vi "Periodic Tasks.vi"   [LabVIEW 2015]
doc: "This VI runs in parallel to other robot code. It can contain as many user-defined periodic loops as you need. These can carry out PID or other sorts of timed response."
uses:
  <vilib>/Rock Robotics/Network Tables/NT Read Boolean.vi
  Robot Global Data.vi
  <vilib>/Rock Robotics/Network Tables/NT Write Boolean.vi
  <vilib>/Rock Robotics/Network Tables/NT Write Number.vi
  Support Code/Team900-VIs/navX Library v2/navX Library v2.lvlib
types:
  T1 = typedef "navX Library v2.lvlib/Z900_navX_DeviceTypeDef.ctl" = cluster{"Interface":cluster{"Protocol":T2, "Update Rate (4Hz-60Hz)":u8, "navX Open TypeDef":variant}, "Notify Packet":refnum<notifier>, "Loop VI Refnum":refnum<vi>, "Ready to Close Occurrence Refnum":refnum<k4>}
  T2 = typedef "navX Library v2.lvlib/Z900_navX_ProtocolTypeDef.ctl" = enum16{"SERIAL", "I2C", "SPI"}
  T3 = cluster{"Yaw":dbl, "Roll":dbl, "Pitch":dbl, "Heading":dbl, "Fused Heading":dbl}
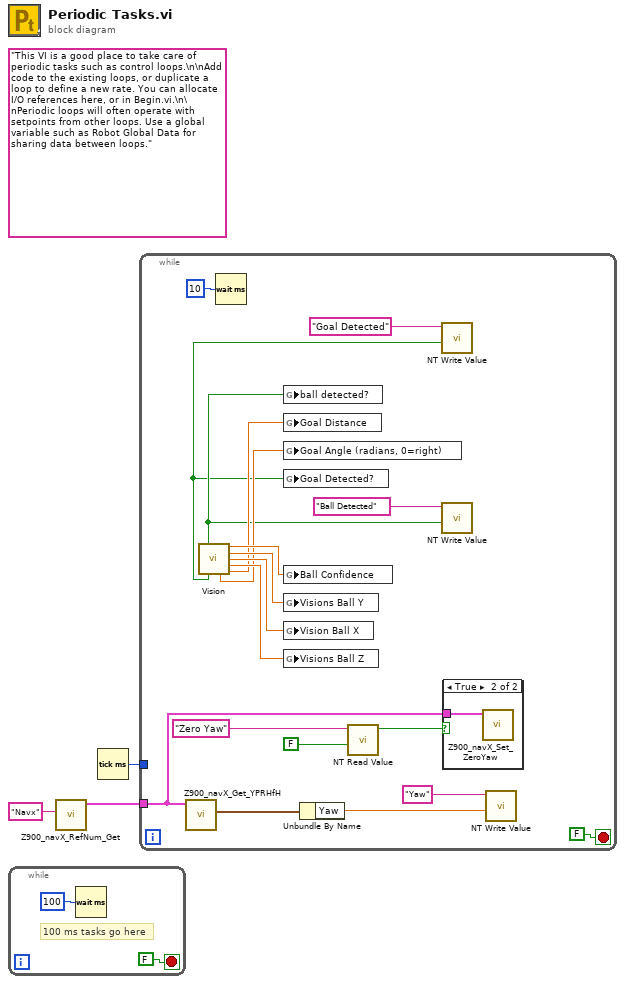
[diagram p0: block diagram]
diagram:
  (unwired) "This VI is a good place to take care of periodic tasks such as control loops.\n\nAdd code to the existing loops, or duplicate a loop to define a new rate. You can allocate I/O references here, or in Begin.vi.\n\nPeriodic loops will often operate with setpoints from other loops. Use a global variable such as Robot Global Data for sharing data between loops."
  n1 = while {
    stop <- FALSE stop-if-true
    # "100 ms tasks go here"
    n2 = Wait (ms)(milliseconds to wait=u32 100) -> ()  [unwired: 1 out]
  }
  n3 = call "Z900_navX_RefNum_Get.vi"("refnum name"="Navx") -> ("navX Device"=w1:T1)  [unwired: 9 in, 1 out]
  n4 = Tick Count (ms)() -> (millisecond timer value=w3:u32)
  n5 = while {
    tunnel: w3 -> [_]
    tunnel: w1 -> [w13]
    stop <- FALSE stop-if-true
    n6 = call "Z900_navX_Get_YPRHfH.vi"("navX Device"=w13) -> ("YRPHfH"=w12:T3)  [unwired: 7 in, 3 out]
    n7 = call "Vision.vi"() -> ("ball detected"=w8:bool, "Confidence"=w22:dbl, "y Coordinate of Ball"=w21:dbl, "x Coordinate of Ball"=w20:dbl, "z Coordinate of Goal"=w19:dbl, "Goal Detected"=w6:bool, "Goal Angle (radians 0=right)"=w17:dbl, "Goal Distance"=w18:dbl)  [unwired: 8 in]
    n8 = Wait (ms)(milliseconds to wait=u32 10) -> ()  [unwired: 1 out]
    n9 = global write "Robot Global Data.vi" "ball detected?"(w8) -> ()
    n10 = global write "Robot Global Data.vi" "Goal Distance"(w18) -> ()
    n11 = global write "Robot Global Data.vi" "Goal Angle (radians, 0=right)"(w17) -> ()
    n12 = global write "Robot Global Data.vi" "Goal Detected?"(w6) -> ()
    n13 = global write "Robot Global Data.vi" "Ball Confidence"(w22) -> ()
    n14 = global write "Robot Global Data.vi" "Visions Ball Y"(w21) -> ()
    n15 = global write "Robot Global Data.vi" "Vision Ball X"(w20) -> ()
    n16 = global write "Robot Global Data.vi" "Visions Ball Z"(w19) -> ()
    n17 = Unbundle By Name(w12) -> ("Yaw"=w10:dbl)
    n18 = call-poly <vilib>:"NT Read Value.vi"("Default Value"=FALSE, "Name"="Zero Yaw") -> ("Boolean"=w16:bool)  [unwired: 8 in, 1 out]
    n19 = call-poly <vilib>:"NT Write Value.vi"("Boolean"=w6, "Name"="Goal Detected") -> ()  [unwired: 9 in, 1 out]
    n20 = call-poly <vilib>:"NT Write Value.vi"("Boolean"=w8, "Name"="Ball Detected") -> ()  [unwired: 9 in, 1 out]
    n21 = case shown="True" w16 {
      tunnel: w13 -> [_ w25]
      frame False {
      }
      frame True {
        n22 = call "Z900_navX_Set_ZeroYaw.vi"("navX Device"=w25) -> ()  [unwired: 9 in, 2 out]
      }
    }
    n23 = call-poly <vilib>:"NT Write Value.vi"("Numeric"=w10, "Name"="Yaw") -> ()  [unwired: 9 in, 1 out]
  }
